vi "CRYAttack-Release Start Search.vi"(8 "Attack? (T)":bool=TRUE, 9 "Filter rank (8)":i32=8, 10 "Init & final avg (16)":i32=16, 11 "Time data in":dbl[](array[numeric]) format="%.2f") -> (3 "Pulse start index":i32)   [LabVIEW 2013]
uses:
  <vilib>/Analysis/NI_AALBase.lvlib
panel:
  # "Attack"
  # "Release"
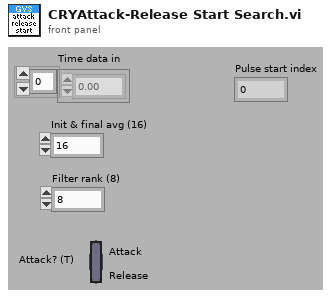
[diagram p1: front panel]
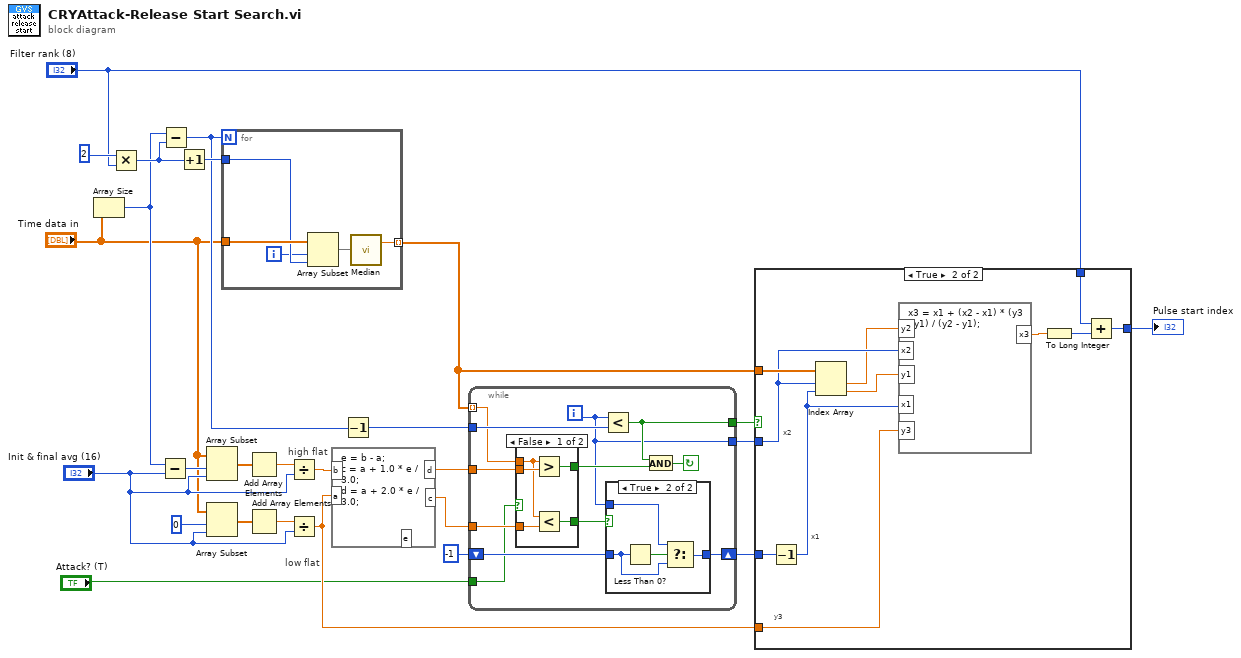
[diagram p0: block diagram]
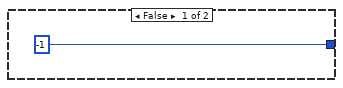
[diagram p2: hidden frame]
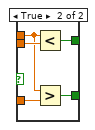
[diagram p3: hidden frame]
diagram:
  # "high flat"
  # "low flat"
  n1 = Array Size(array="Time data in") -> (size(s)=w23:i32)
  n2 = Multiply(x=2, y="Filter rank (8)") -> (x*y=w25:i32)
  n3 = Subtract(x=w23, y="Init & final avg (16)") -> (x-y=w22:i32)
  n4 = Subtract(x=w23, y=w25) -> (x-y=w15:i32)
  n5 = Increment(x=w25) -> (x+1=w24:i32)
  n6 = Array Subset(array="Time data in", index=w22, length="Init & final avg (16)") -> (w20:dbl[])
  n7 = Array Subset(array="Time data in", index=0 ("Array Index"), length="Init & final avg (16)") -> (w18:dbl[])
  n8 = for {
    N: w15 -> [_]
    tunnel: "Time data in" -> [w31]
    tunnel: w24 -> [w30]
    tunnel: [w28] -> w11 mode=indexing
    i -> [w27]
    n9 = Array Subset(array=w31, index=w27, length=w30) -> (w29:dbl[])
    n10 = call <vilib>:"Median.vi"("X"=w29) -> ("median"=w28:dbl)  [unwired: 1 out]
  }
  n11 = Add Array Elements(numeric array=w20) -> (sum=w19:dbl)
  n12 = Add Array Elements(numeric array=w18) -> (sum=w17:dbl)
  n13 = Divide(x=w19, y="Init & final avg (16)") -> (x/y=w8:dbl)
  n14 = Divide(x=w17, y="Init & final avg (16)") -> (x/y=w5:dbl)
  n15 = formula code="e = b - a;\nc = a + 1.0 * e / 3.0;\nd = a + 2.0 * e / 3.0;"("b"=w8, "a"=w5) -> ("d"=w6:dbl, "c"=w7:dbl)  [unwired: 1 out]
  n16 = Decrement(x=w15) -> (x-1=w14:i32)
  n17 = while {
    tunnel: w11 -> [w33] mode=indexing
    tunnel: w14 -> [w39]
    tunnel: w7 -> [w43]
    tunnel: w6 -> [w38]
    shift-right: [w40] -> w9
    shift-left: -1 -> [w41]
    tunnel: [w34] -> w10
    tunnel: [w35] -> w12
    tunnel: "Attack? (T)" -> [w32]
    i -> [w34]
    stop <- w36 continue-if-true
    n18 = case shown="False" w32 {
      tunnel: w43 -> [w48 w53]
      tunnel: [w47 w52] -> w42
      tunnel: w38 -> [w46 w51]
      tunnel: [w45 w50] -> w37
      tunnel: w33 -> [w44 w49]
      frame False {
        n19 = Greater?(x=w44, y=w46) -> (0:w45:bool)
        n20 = Less?(x=w44, y=w48) -> (x < y?=w47:bool)
      }
      frame True {
        n21 = Less?(x=w49, y=w51) -> (x < y?=w50:bool)
        n22 = Greater?(x=w49, y=w53) -> (0:w52:bool)
      }
    }
    n23 = Less?(x=w34, y=w39) -> (x < y?=w35:bool)
    n24 = case shown="True" w42 {
      tunnel: w41 -> [w54 w56]
      tunnel: w34 -> [_ w57]
      tunnel: [w54 w55] -> w40
      frame False {
      }
      frame True {
        n25 = Less Than 0?(x=w56) -> (x < 0?=w58:bool)
        n26 = Select(t=w57, s=w58, f=w56) -> (s? t:f=w55:i32)
      }
    }
    n27 = And(x=w35, y=w37) -> (x .and. y?=w36:bool)
  }
  n28 = case shown="True" w12 {
    tunnel: w11 -> [_ w69]
    tunnel: w10 -> [_ w68]
    tunnel: w9 -> [_ w70]
    tunnel: w5 -> [_ w64]
    tunnel: [-1 w60] -> w4
    tunnel: "Filter rank (8)" -> [_ w62]
    frame False {
    }
    frame True {
      # "y3"
      # "x2"
      # "x1"
      n29 = Decrement(x=w70) -> (x-1=w65:i32)
      n30 = Index Array(array=w69, index #1=w68, index #2=w65) -> (element #1=w67:dbl, element #2=w66:dbl)
      n31 = formula code="x3 = x1 + (x2 - x1) * (y3 - y1) / (y2 - y1);"("y2"=w67, "x2"=w68, "y1"=w66, "x1"=w65, "y3"=w64) -> ("x3"=w63:dbl)
      n32 = To Long Integer(number=w63) -> (32bit integer=w61:i32)
      n33 = Add(x=w62, y=w61) -> (x+y=w60:i32)
    }
  }
  "Pulse start index" <- w4
